vi "Read Payload.vi"(8 "error in":errorcluster, 11 "CutomOOB_Tx in":refnum<class "TemplateOOB_Tx.lvclass">) -> (0 "error out":errorcluster, 2 "data":T1, 3 "CutomOOB_Tx out":refnum<class "TemplateOOB_Tx.lvclass">)   [LabVIEW 2021, in "TemplateOOB_Tx.lvclass"]
uses:
  TemplateOOB_Tx.lvclass
  D:/dev/CIF-LVCore/src/CIFUtilities/CIFOutOfBand/CIFOutOfBand.lvclass
  Typedef/Payload.ctl
  Typedef/Main to gRPC Command Data.ctl
  CIF-LVCore/src/CIFUtilities/CIFOutOfBand/CIFOutOfBand.lvclass/CIFOutOfBand.ctl
  TemplateOOB_Tx.lvclass/TemplateOOB_Tx.ctl
  CIF-LVCore/src/CIFUtilities/CIFOutOfBand/CIFOutOfBand.lvclass
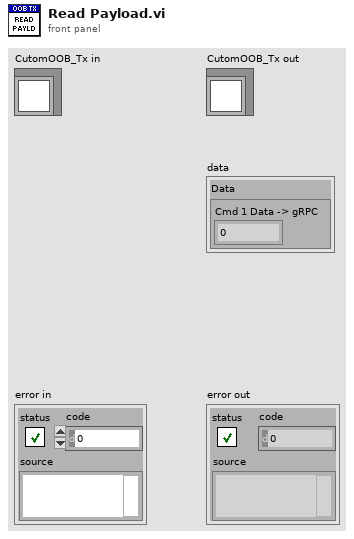
[diagram p1: front panel]
types:
  T1 = typedef "TemplateOOB_Tx.lvclass/Payload.ctl" = cluster{"Data":T2}
  T2 = typedef "TemplateOOB_Tx.lvclass/Main to gRPC Command Data.ctl" = cluster{"Cmd 1 Data -> gRPC":i32}
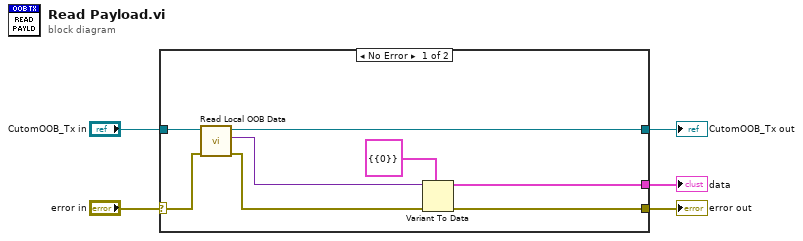
[diagram p0: block diagram]
diagram:
  n1 = case shown="No Error" "error in" {
    selector: "error in" -> [w12 w15]
    tunnel: [w11 w15] -> w5
    tunnel: [w7 w14] -> w4
    tunnel: "CutomOOB_Tx in" -> [w13 w14]
    tunnel: [w6 _] -> w1
    frame No Error {
      n2 = call "Read Local OOB Data.vi"("error in"=w12, "OOB in"=w13) -> ("error out"=w10:errorcluster, "Local OOB Data"=w9:variant, "OOB out"=w7:refnum<class "TemplateOOB_Tx.lvclass">)  [unwired: 7 in]
      n3 = Variant To Data(error in=w10, type=T1 {"Data"={"Cmd 1 Data -> gRPC"=0}}, Variant=w9) -> (data=w6:T1, error out=w11:errorcluster)
    }
    frame Error {
    }
  }
  "error out" <- w5
  "CutomOOB_Tx out" <- w4
  "data" <- w1
